vi "Oscilloscope.vi"() -> ()   [LabVIEW 2016]
uses:
  QSM-PC (String)/Library/QSM-PC (String).lvlib
panel:
  out "percent":dbl
  in  "元素":cluster{"State":string, "Data":variant}
  out "State":string
  out "波形图":dbl[][](graph)
  out "QSM - Oscilloscope":refnum<queue>
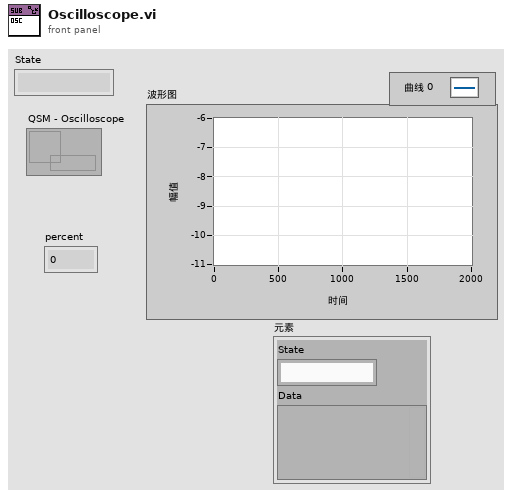
[diagram p1: front panel]
types:
  T1 = cluster{"Type":string, "percent":dbl, "Dev":string}
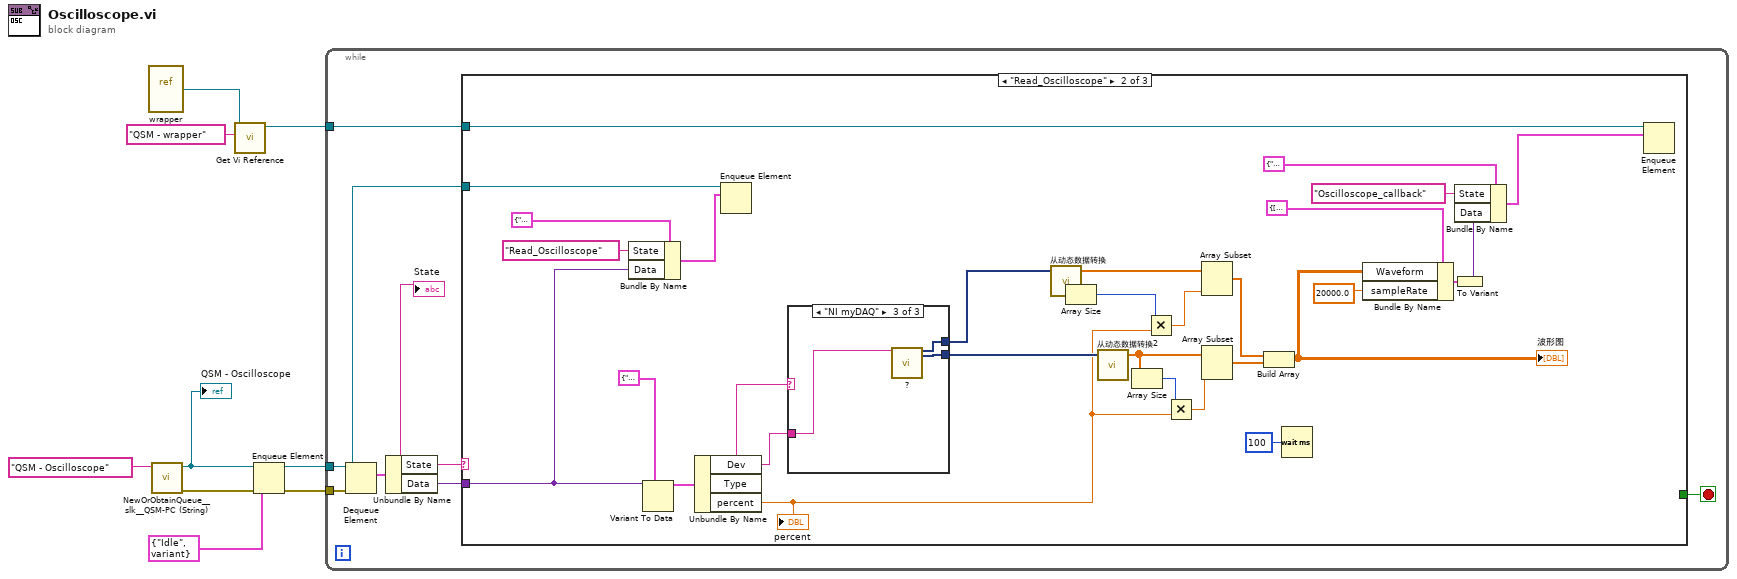
[diagram p0: block diagram]
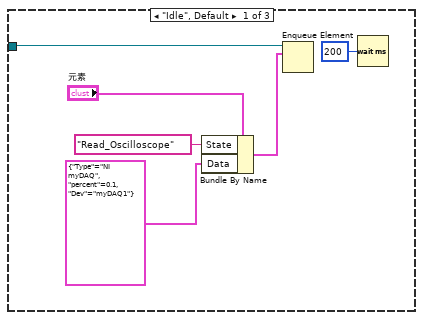
[diagram p2: hidden frame]
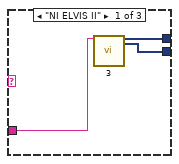
[diagram p3: hidden frame]
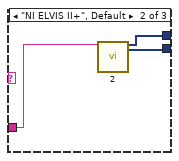
[diagram p4: hidden frame]
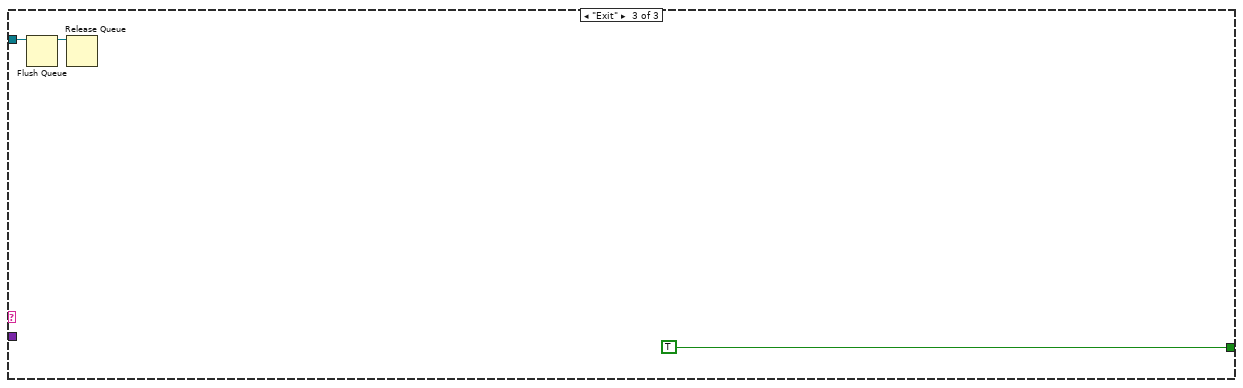
[diagram p5: hidden frame]
diagram:
  n1 = vi-ref "wrapper.vi"() -> (w2:refnum<vi>)
  n2 = call "NewOrObtainQueue__slk__QSM-PC (String).vi"("queue name in"="QSM - Oscilloscope") -> ("error out"=w7:errorcluster, "queue out"=w8:refnum<queue>)  [unwired: 2 in, 7 out]
  "QSM - Oscilloscope" <- w8
  n3 = call "Get Vi Reference.vi"("Control name"="QSM - wrapper", "Vi Reference in"=w2) -> ("队列输出"=w9:refnum<queue>)  [unwired: 6 in, 2 out]
  n4 = Enqueue Element(queue=w8, element=cluster{"State":string, "Data":variant} {"State"="Idle", "Data"=variant} ("元素"), error in (no error)=w7) -> (queue out=w5:refnum<queue>, error out=w3:errorcluster)  [unwired: 2 out]
  n5 = while {
    tunnel: w9 -> [w15]
    tunnel: w5 -> [w14]
    tunnel: w3 -> [w10]
    stop <- w13 stop-if-true
    n6 = Dequeue Element(queue=w14, error in (no error)=w10) -> (element=w12:cluster{"State":string, "Data":variant})  [unwired: 1 in, 3 out]
    n7 = Unbundle By Name(w12) -> ("State"=w11:string, "Data"=w16:variant)
    "State" <- w11
    n8 = case shown="\"Read_Oscilloscope\"" w11 {
      tunnel: w16 -> [_ w25 _]
      tunnel: w15 -> [_ w41 _]
      tunnel: w14 -> [w21 w40 w64]
      tunnel: [_ _ TRUE] -> w13
      frame "Idle", Default {
        n9 = Bundle By Name(cluster="元素", "State"="Read_Oscilloscope", "Data"=T1 {"Type"="NI myDAQ", "percent"=0.1, "Dev"="myDAQ1"}) -> (w18:cluster{"State":string, "Data":variant})
        n10 = Enqueue Element(queue=w21, element=w18) -> ()  [unwired: 2 in, 3 out]
        n11 = Wait (ms)(milliseconds to wait=u32 200 ("等待时间（毫秒）")) -> ()  [unwired: 1 out]
      }
      frame "Read_Oscilloscope" {
        n12 = Bundle By Name(cluster=cluster{"State":string, "Data":variant} {"State"="", "Data"=variant} ("元素"), "State"="Read_Oscilloscope", "Data"=w25) -> (w27:cluster{"State":string, "Data":variant})
        n13 = Variant To Data(type=T1 {"Type"="", "percent"=0.0, "Dev"=""}, Variant=w25) -> (data=w23:T1)  [unwired: 1 in, 1 out]
        n14 = Unbundle By Name(w23) -> ("Dev"=w29:string, "Type"=w30:string, "percent"=w42:dbl)
        "percent" <- w42
        n15 = Enqueue Element(queue=w40, element=w27) -> ()  [unwired: 2 in, 3 out]
        n16 = case shown="\"NI myDAQ\"" w30 {
          tunnel: [w54 w58 w61] -> w46
          tunnel: [w55 w57 w60] -> w45
          tunnel: w29 -> [w53 w56 w59]
          frame "NI ELVIS II" {
            n17 = call "3"("Device Name"=w53) -> ("ELVIS/Channel 0"=w55:dynamicdata, "ELVIS/Channel 1"=w54:dynamicdata)  [unwired: 16 in, 1 out]
          }
          frame "NI ELVIS II+", Default {
            n18 = call "2"("Device Name"=w56) -> ("ELVIS/Channel 0"=w57:dynamicdata, "ELVIS/Channel 1"=w58:dynamicdata)  [unwired: 16 in, 1 out]
          }
          frame "NI myDAQ" {
            n19 = call "?"("Device Name"=w59) -> ("myDAQ/Channel 0"=w60:dynamicdata, "myDAQ/Channel 1"=w61:dynamicdata)  [unwired: 16 in, 1 out]
          }
        }
        n20 = call "从动态数据转换"("Dynamic Data Type"=w45) -> ("Array"=w52:dbl[])  [unwired: 3 in]
        n21 = Array Size(array=w52) -> (size(s)=w51:i32)
        n22 = call "从动态数据转换2"("Dynamic Data Type"=w46) -> ("Array"=w47:dbl[])  [unwired: 3 in]
        n23 = Array Size(array=w47) -> (size(s)=w48:i32)
        n24 = Multiply(x=w51, y=w42) -> (x*y=w50:dbl)
        n25 = Multiply(x=w48, y=w42) -> (x*y=w49:dbl)
        n26 = Array Subset(array=w52, length=w50) -> (w44:dbl[])  [unwired: 1 in]
        n27 = Array Subset(array=w47, length=w49) -> (w43:dbl[])  [unwired: 1 in]
        n28 = Build Array(w44, w43) -> (w38:dbl[][])
        "波形图" <- w38
        n29 = Wait (ms)(milliseconds to wait=u32 100 ("等待时间（毫秒）")) -> ()  [unwired: 1 out]
        n30 = Bundle By Name(cluster=cluster{"Waveform":dbl[][], "sampleRate":dbl} {"Waveform"=[], "sampleRate"=0.0}, "Waveform"=w38, "sampleRate"=20000.0) -> (w32:cluster{"Waveform":dbl[][], "sampleRate":dbl})
        n31 = To Variant(anything=w32) -> (Variant=w33:variant)
        n32 = Bundle By Name(cluster=cluster{"State":string, "Data":variant} {"State"="", "Data"=variant} ("元素"), "State"="Oscilloscope_callback", "Data"=w33) -> (w37:cluster{"State":string, "Data":variant})
        n33 = Enqueue Element(queue=w41, element=w37) -> ()  [unwired: 2 in, 3 out]
      }
      frame "Exit" {
        n34 = Flush Queue(queue=w64) -> (queue out=w62:refnum<queue>)  [unwired: 1 in, 2 out]
        n35 = Release Queue(queue=w62) -> ()  [unwired: 2 in, 3 out]
      }
    }
  }
